vi "Get TreeItem Parent Indices.vi"(10 "TreeItem Index":i32, 11 "TreeItems":T1[](array[typedef])) -> (2 "TreeItem index indent":i32, 3 "parent indices (incrementing)":i32[](array[numeric]))   [LabVIEW 2020, in "BetterDragAndDrop.lvlib" / "BetterTreeHandle.lvclass"]
uses:
  Classes/BetterTreeHandle/BetterTreeHandle.lvclass
  Classes/BetterTreeItem/SubVIs/TreeItem.ctl
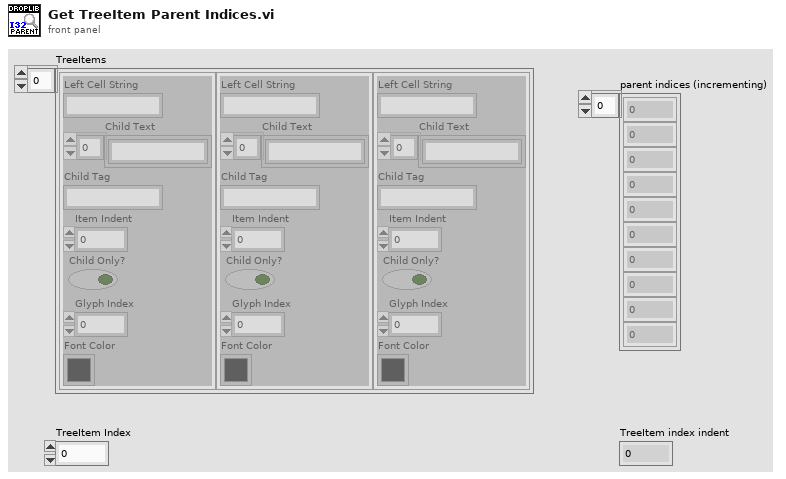
[diagram p1: front panel]
types:
  T1 = typedef "BetterDragAndDrop.lvlib/BetterTreeHandle.lvclass/TreeItem.ctl" = cluster{"Left Cell String":string, "Child Text":string[], "Child Tag":string, "Item Indent":i32, "Child Only?":bool, "Glyph Index":i32, "Font Color":u32}
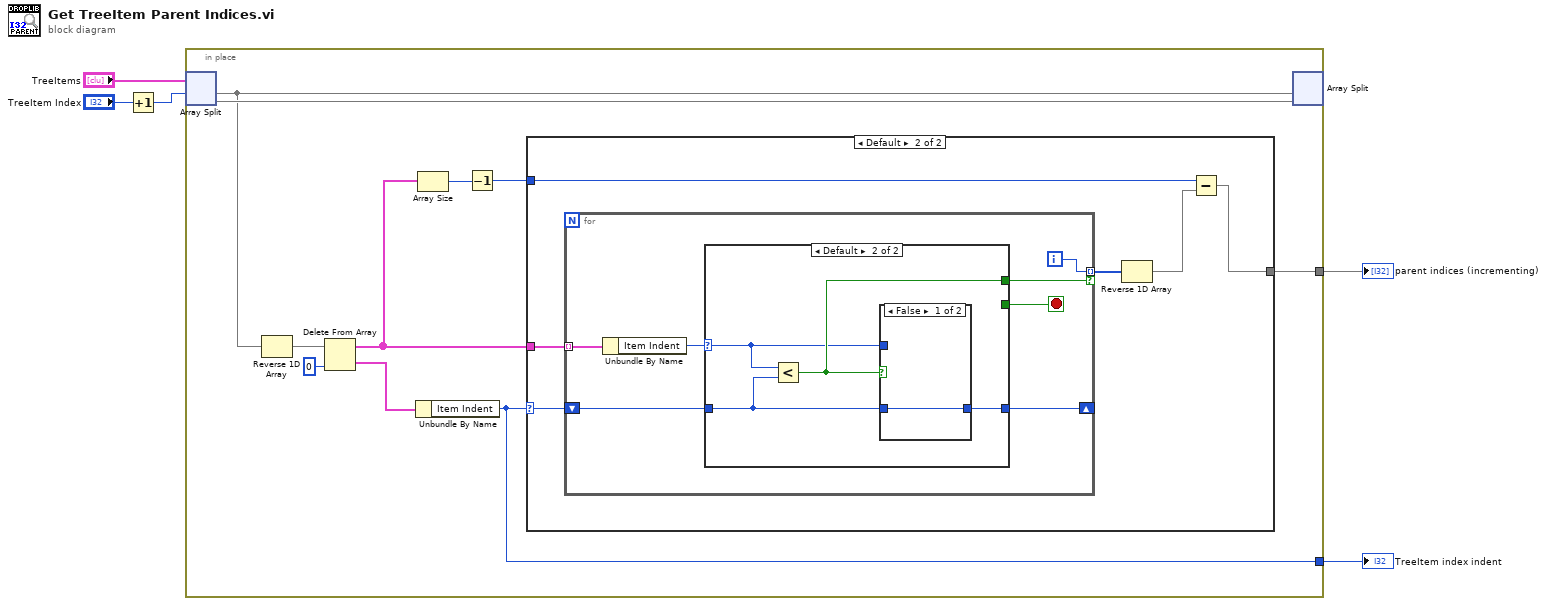
[diagram p0: block diagram]
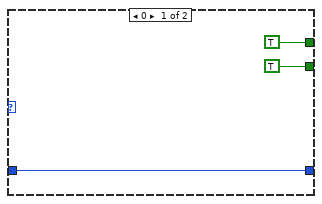
[diagram p3: hidden frame]
diagram:
  n1 = Increment(x="TreeItem Index") -> (x+1=w1:i32)
  n2 = in-place {
    in-place-border: [w13] -> w4
    in-place-border: [w12] -> w3
    n3 = in-place-split #1("TreeItems", w1) -> (w14:T1[], w15:T1[])
    n4 = Reverse 1D Array(array=w14) -> (reversed array=w11:T1[])
    n5 = Delete From Array(array=w11, index=0) -> (deleted portion=w9:T1, array with subset deleted=w8:T1[])  [unwired: 1 in]
    n6 = Unbundle By Name(w9) -> ("Item Indent"=w12:i32)
    n7 = Array Size(array=w8) -> (size(s)=w7:i32)
    n8 = Decrement(x=w7) -> (x-1=w6:i32)
    n9 = case shown="Default" w12 {
      selector: w12 -> [_ w21]
      tunnel: w8 -> [_ w20]
      tunnel: [_ w19] -> w13
      tunnel: w6 -> [_ w18]
      frame 0 {
      }
      frame Default {
        n10 = for {
          tunnel: w20 -> [w28] mode=indexing
          shift-right: [w24] -> _
          shift-left: w21 -> [w23]
          tunnel: [w27] -> w17 mode=indexing if=w26
          i -> [w27]
          stop <- w22 stop-if-true
          n11 = Unbundle By Name(w28) -> ("Item Indent"=w25:i32)
          n12 = case shown="Default" w25 {
            selector: w25 -> [_ w34]
            tunnel: [TRUE w35] -> w26
            tunnel: [w30 w33] -> w24
            tunnel: w23 -> [w30 w32]
            tunnel: [TRUE _] -> w22
            frame 0 {
            }
            frame Default {
              n13 = Less?(x=w34, y=w32) -> (x < y?=w35:bool)
              n14 = case shown="False" w35 {
                tunnel: w34 -> [_ w37]
                tunnel: [w36 w37] -> w33
                tunnel: w32 -> [w36 _]
                frame False {
                }
                frame True {
                }
              }
            }
          }
        }
        n15 = Reverse 1D Array(array=w17) -> (reversed array=w16:i32[])
        n16 = Subtract(x=w18, y=w16) -> (x-y=w19:i32[])
      }
    }
    n17 = in-place-split #1(w14, w15) -> ()  [unwired: 2 out]
  }
  "parent indices (incrementing)" <- w4
  "TreeItem index indent" <- w3
